vi "assemble.vi"(8 "error in (no error)":errorcluster, 11 "Furniture in":refnum<class "Furniture.lvclass">) -> (0 "error out":errorcluster, 2 "String":string, 3 "Furniture out":refnum<class "Furniture.lvclass">)   [LabVIEW 2021, in "Furniture.lvclass"]
uses:
  Furniture.lvclass
  Furniture.lvclass/Furniture.ctl
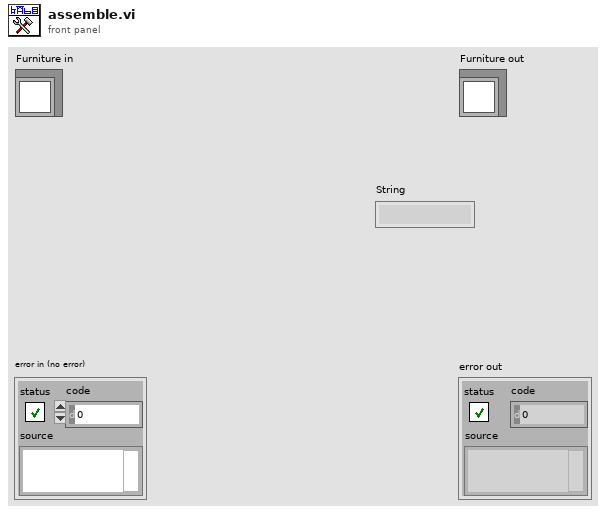
[diagram p1: front panel]
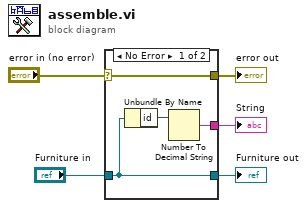
[diagram p0: block diagram]
diagram:
  n1 = case shown="No Error" "error in (no error)" {
    selector: "error in (no error)" -> [w9 w11]
    tunnel: [w9 w11] -> w4
    tunnel: [w8 w10] -> w2
    tunnel: "Furniture in" -> [w8 w10]
    tunnel: [w6 _] -> w1
    frame No Error {
      n2 = Unbundle By Name(w8) -> ("id"=w7:u32)
      n3 = Number To Decimal String(number=w7) -> (decimal integer string=w6:string)  [unwired: 1 in]
    }
    frame Error {
    }
  }
  "error out" <- w4
  "Furniture out" <- w2
  "String" <- w1
